vi "Calculate_PID_Output(SubVI).vi"(6 "Condition":bool, 7 "PID_Discrete_In":T2, 8 "X k-2":dbl, 9 "X k-1":dbl, 10 "X k":dbl, 11 "Y k-1":dbl) -> (2 "Y k":dbl)   [LabVIEW 2017]
uses:
  PID_Discrete_Coefficients.ctl
  Controller_Type.ctl
panel:
  in  "Controller type":T1
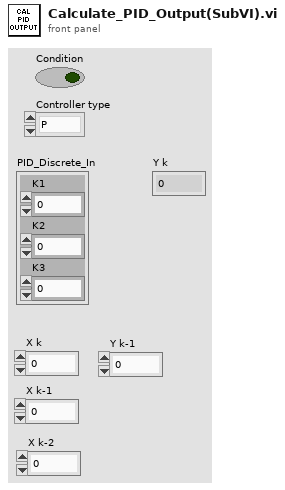
[diagram p1: front panel]
types:
  T1 = typedef "Controller_Type.ctl" = enum16{"P", "PI", "PD", "PID"}
  T2 = typedef "PID_Discrete_Coefficients.ctl" = cluster{"K1":dbl, "K2":dbl, "K3":dbl}
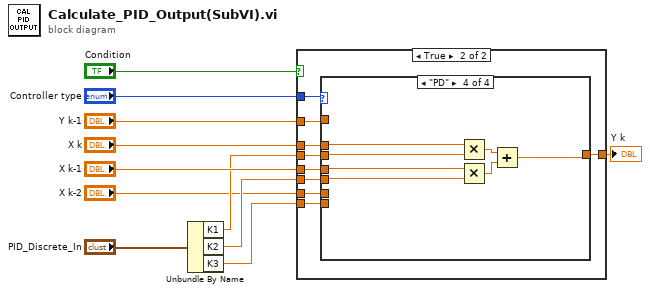
[diagram p0: block diagram]
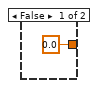
[diagram p2: hidden frame]
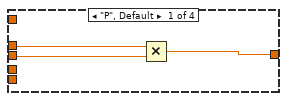
[diagram p3: hidden frame]
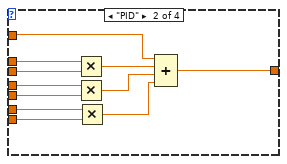
[diagram p4: hidden frame]
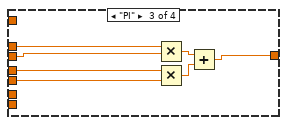
[diagram p5: hidden frame]
diagram:
  n1 = Unbundle By Name("PID_Discrete_In") -> ("K1"=w5:dbl, "K2"=w6:dbl, "K3"=w4:dbl)
  n2 = case shown="True" "Condition" {
    tunnel: "Y k-1" -> [_ w21]
    tunnel: [0.0 w20] -> w10
    tunnel: "X k-1" -> [_ w19]
    tunnel: "X k" -> [_ w18]
    tunnel: w6 -> [_ w17]
    tunnel: w5 -> [_ w16]
    tunnel: w4 -> [_ w15]
    tunnel: "X k-2" -> [_ w14]
    tunnel: "Controller type" -> [_ w13]
    frame False {
    }
    frame True {
      n3 = case shown="\"PD\"" w13 {
        tunnel: w21 -> [_ w35 _ _]
        tunnel: [w22 w34 w36 w47] -> w20
        tunnel: w19 -> [_ w33 w41 w44]
        tunnel: w18 -> [w24 w32 w38 w46]
        tunnel: w17 -> [_ w28 w40 w43]
        tunnel: w16 -> [w23 w27 w37 w45]
        tunnel: w15 -> [_ w26 _ _]
        tunnel: w14 -> [_ w25 _ _]
        frame "P", Default {
          n4 = Multiply(x=w24, y=w23) -> (x*y=w22:dbl)
        }
        frame "PID" {
          n5 = Multiply(x=w32, y=w27) -> (x*y=w29:dbl)
          n6 = Multiply(x=w33, y=w28) -> (x*y=w31:dbl)
          n7 = Multiply(x=w25, y=w26) -> (x*y=w30:dbl)
          n8 = Compound Arithmetic op=ADD(w35, w29, w31, w30) -> (w34:dbl)
        }
        frame "PI" {
          n9 = Multiply(x=w38, y=w37) -> (x*y=w39:dbl)
          n10 = Multiply(x=w41, y=w40) -> (x*y=w42:dbl)
          n11 = Add(x=w39, y=w42) -> (x+y=w36:dbl)
        }
        frame "PD" {
          n12 = Multiply(x=w46, y=w45) -> (x*y=w48:dbl)
          n13 = Multiply(x=w44, y=w43) -> (x*y=w49:dbl)
          n14 = Add(x=w48, y=w49) -> (x+y=w47:dbl)
        }
      }
    }
  }
  "Y k" <- w10
